vi "Get Initially Connected Endpoints.vi"(8 "error in (no error)":errorcluster, 11 "Hardware Ref in":T2 format="%.0x") -> (0 "error out":errorcluster, 2 "Connections":T1[](array[typedef]), 3 "Hardware Ref out":T2 format="%.0x")   [LabVIEW 2017, in "Routing and Faulting Hardware API.lvlib"]
uses:
  Routing and Faulting Hardware API.lvlib
  <vilib>/NI Veristand/Custom Device API/Custom Device Item Ref.ctl
  Types/Connection.ctl
  Routing and Faulting Hardware API Constants.vi
  <vilib>/NI Veristand/Custom Device API/Get Item Property (String Array).vi
  <vilib>/regexp/Match Regular Expression.xnode
  <vilib>/NI Veristand/Custom Device API/Custom Device API.lvlib
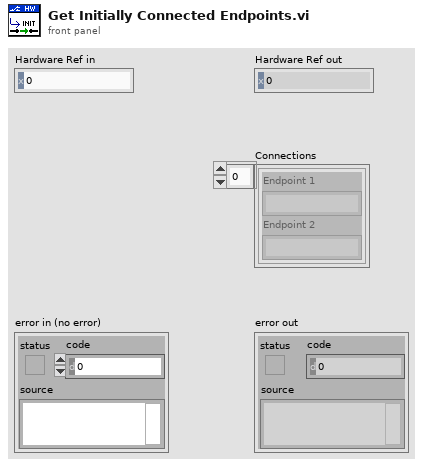
[diagram p1: front panel]
types:
  T1 = typedef "Routing and Faulting Hardware API.lvlib/Connection.ctl" = cluster{"Endpoint 1":string, "Endpoint 2":string}
  T2 = typedef "Custom Device API.lvlib/Custom Device Item Ref.ctl" = u64
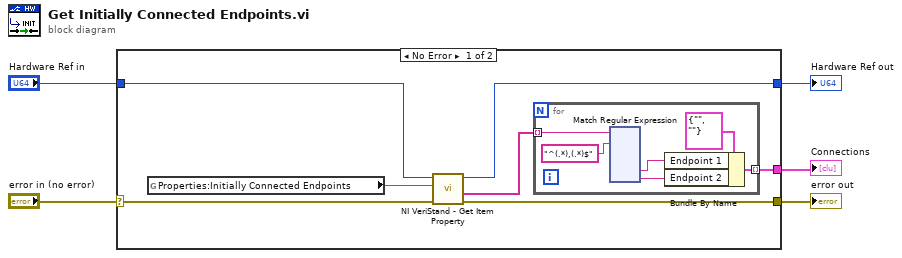
[diagram p0: block diagram]
diagram:
  n1 = case shown="No Error" "error in (no error)" {
    selector: "error in (no error)" -> [w9 w137]
    tunnel: "Hardware Ref in" -> [w12 w136]
    tunnel: [w11 w136] -> w4
    tunnel: [w10 w137] -> w3
    tunnel: [w6 _] -> w1
    frame No Error {
      n2 = global read "Routing and Faulting Hardware API Constants.vi" "Properties:Initially Connected Endpoints"() -> (w8:string)
      n3 = call-poly <vilib>:"NI VeriStand - Get Item Property.vi"("error in (no error)"=w9, "Property Name"=w8, "Item Ref in"=w12) -> ("error out"=w10:errorcluster, "Value"=w7:string[], "Item Ref out"=w11:T2)  [unwired: 5 in, 1 out]
      n4 = for {
        tunnel: w7 -> [w17] mode=indexing
        tunnel: [w13] -> w6 mode=indexing
        n5 = xnode "Match Regular Expression"("input string"=w17, "regular expression"="^(.*),(.*)$" ("search string")) -> ("submatch 1"=w15:string, "submatch 2"=w14:string)  [unwired: 4 in, 5 out]
        n6 = Bundle By Name(cluster=T1 {"Endpoint 1"="", "Endpoint 2"=""} ("Connection"), "Endpoint 1"=w15, "Endpoint 2"=w14) -> (w13:T1)
      }
    }
    frame Error {
    }
  }
  "Hardware Ref out" <- w4
  "error out" <- w3
  "Connections" <- w1
